vi "Temp Path.vi"(8 "error in (no error)":errorcluster) -> (0 "error out":errorcluster, 3 "path":path)   [LabVIEW 2026, in "PXI_Common.lvlib"]
uses:
  PXI_Common.lvlib
  <vilib>/Utility/sysdir.llb/System Directory Type.ctl
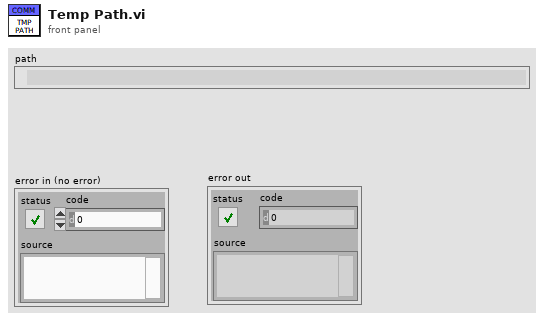
[diagram p1: front panel]
types:
  T1 = enum32{"invalid app kind", "Development System", "Run Time System", "Student Edition", "Embedded LabVIEW", "Evaluation", "Custom"}
  T2 = typedef "System Directory Type.ctl" = i32
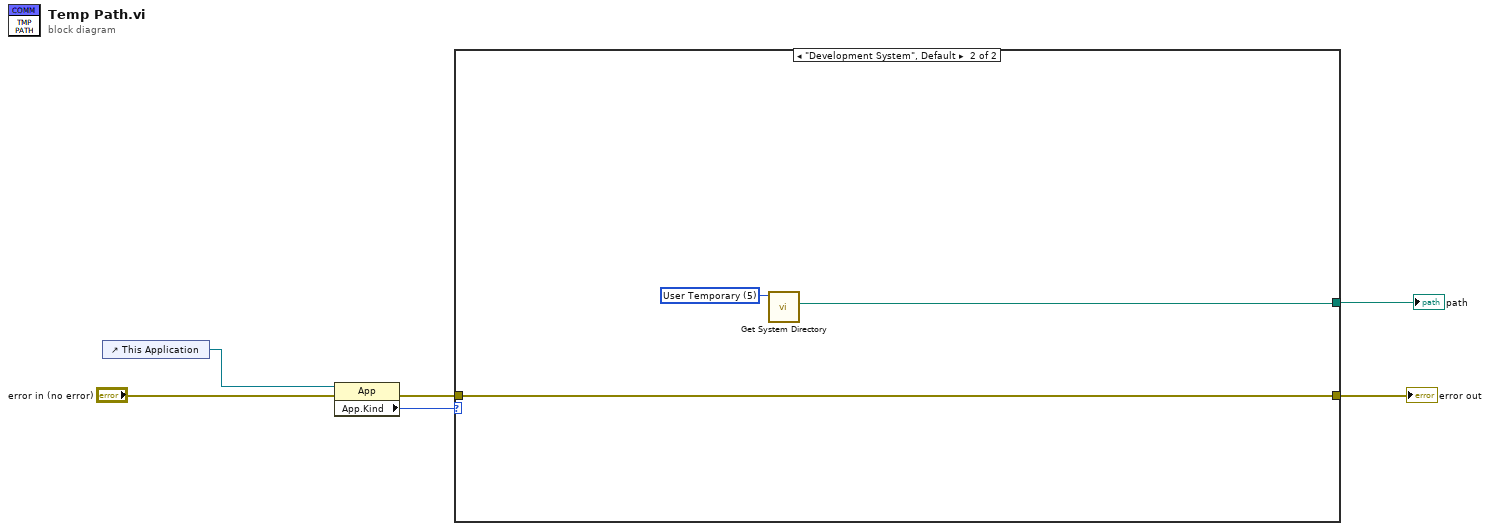
[diagram p0: block diagram]
diagram:
  n1 = control-ref of="This Application"() -> (w5:refnum<vi>)
  n2 = property class="App"(reference=w5, error in="error in (no error)") -> (error out=w3:errorcluster, "App.Kind"=w4:T1)  [unwired: 1 out]
  n3 = case shown="\"Development System\", Default" w4 {
    tunnel: w3 -> [w7 w10]
    tunnel: [_ w9] -> w2
    tunnel: [w7 w10] -> w1
    frame "Run Time System" {
    }
    frame "Development System", Default {
      w8 = T2 5 items=["User Home"=0, "User Desktop"=1, "User Documents"=2, "User Application Data"=3, "User Preferences"=4, "User Temporary"=5, "Public Documents"=6, "Public Application Data"=7, "Public Preferences"=8, "Public Cache"=13, "System Core Libraries"=9, "System Installed Libraries"=10, "Application Files"=11, "Boot Volume Root"=12] ("system directory type")
      n4 = call <vilib>:"Get System Directory.vi"("system directory type"=w8) -> ("system directory"=w9:path)  [unwired: 10 in]
    }
  }
  "error out" <- w1
  "path" <- w2
